vi "Get Core Reference.vi"(8 "error in (no error)":errorcluster, 11 "Halfwave Fit Display in":refnum<class "Halfwave Fit Display.lvclass">) -> (0 "error out":errorcluster, 2 "Core Ref":refnum<vi>, 3 "Halfwave Fit Display out":refnum<class "Halfwave Fit Display.lvclass">)   [LabVIEW 2016, in "Halfwave Fit Display.lvclass"]
uses:
  Halfwave Fit Display.lvclass
  Sinusoidal Fit/Sinusoidal Fit.lvclass
  Halfwave Fit Display.lvclass/Halfwave Fit Display.ctl
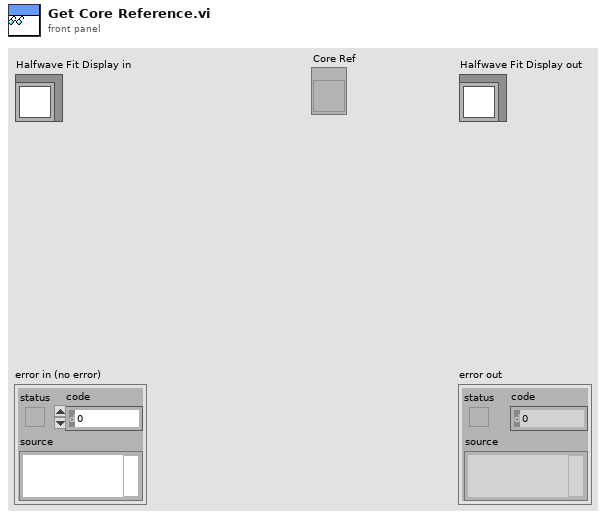
[diagram p1: front panel]
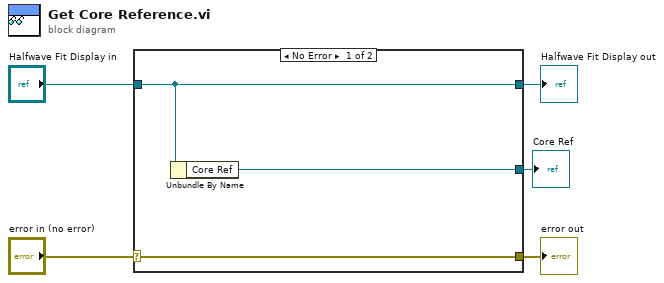
[diagram p0: block diagram]
diagram:
  n1 = case shown="No Error" "error in (no error)" {
    selector: "error in (no error)" -> [w8 w9]
    tunnel: [w8 w9] -> w4
    tunnel: [w7 w10] -> w2
    tunnel: "Halfwave Fit Display in" -> [w7 w10]
    tunnel: [w6 _] -> w1
    frame No Error {
      n2 = Unbundle By Name(w7) -> ("Core Ref"=w6:refnum<vi>)
    }
    frame Error {
    }
  }
  "error out" <- w4
  "Halfwave Fit Display out" <- w2
  "Core Ref" <- w1
